vi "Periodic Tasks.vi"(8 "error in":errorcluster) -> ()   [LabVIEW 2013]
doc: "This VI runs in parallel to other tasks. It can contain as many user-defined periodic loops as you need. These can carry out PID or other sorts of timed response."
uses:
  <vilib>/Rock Robotics/SystemInterfaces/Utilities/FPGA_UtilitiesLED Source.ctl
  <vilib>/Rock Robotics/SystemInterfaces/Utilities/FPGA_UtilitiesLED State.ctl
  <vilib>/Rock Robotics/WPI/Solenoid/WPI_SolenoidValue.ctl
  Robot Global Data.vi
  <vilib>/Rock Robotics/WPI/Solenoid/WPI_SolenoidSetEnum.vi
  <vilib>/Rock Robotics/WPI/Compressor/WPI_CompressorGetSetRefNum.vi
  <vilib>/Rock Robotics/WPI/RobotDrive/WPI_RobotDriveGetSetRefNum.vi
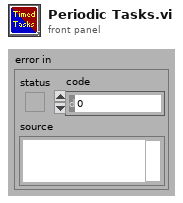
[diagram p1: front panel]
types:
  T1 = typedef "FPGA_UtilitiesLED State.ctl" = enum16{"Off", "On", "Toggle"}
  T2 = typedef "FPGA_UtilitiesLED Source.ctl" = enum16{"User LED", "FPGA LED"}
  T3 = typedef "WPI_CompressorDevRef.ctl" = cluster{"DevStatus":errorcluster, "DigitalInputDevRef":T4, "RelayDevRef":T7}
  T4 = typedef "WPI_DigitalInputDevRef.ctl" = cluster{"DevStatus":errorcluster, "DIO Channel":T5, "Digital Module":T6}
  T5 = typedef "FPGA_DIOChannel.ctl" = enum8{"DIO 1", "DIO 2", "DIO 3", "DIO 4", "DIO 5", "DIO 6", "DIO 7", "DIO 8", "DIO 9", "DIO 10", "DIO 11", "DIO 12", "DIO 13", "DIO 14", "Invalid"}
  T6 = typedef "FPGA_TypedefDigitalModule.ctl" = enum16{"Digital Module 1", "Digital Module 2"}
  T7 = typedef "WPI_RelayDevRef.ctl" = cluster{"DevStatus":errorcluster, "Relay Channel":T8, "Digital Module":T6, "Relay Direction":T9}
  T8 = typedef "FPGA_DIORelayChannel.ctl" = enum8{"Relay 1", "Relay 2", "Relay 3", "Relay 4", "Relay 5", "Relay 6", "Relay 7", "Relay 8", "Invalid"}
  T9 = typedef "WPI_RelayDirection.ctl" = enum16{"Both directions", "Forward only", "Reverse only"}
  T10 = typedef "WPI_RobotDriveDevRef.ctl" = cluster{"DevStatus":errorcluster, "Motors[]":T11[], "Square Inputs":bool, "Max Output":dbl, "Isochronous":bool}
  T11 = typedef "WPI_MotorControlDeviceRef.ctl" = cluster{"DeviceStatus":errorcluster, "Type":enum16{"PWM", "CAN"}, "PWM":cluster{"Digital Module":T6, "PWM Channel":T12, "DeadBand":T13}, "CAN":cluster{"Device Number":u8, "Control Mode":T14, "Semaphore":T15, "Max Vout":dbl}, "Invert":bool, "TransformRef":T16, "InvTransformRef":T16}
  T12 = typedef "FPGA_DIOPWMChannel.ctl" = enum8{"PWM 1", "PWM 2", "PWM 3", "PWM 4", "PWM 5", "PWM 6", "PWM 7", "PWM 8", "PWM 9", "PWM 10", "Invalid"}
  T13 = typedef "WPI_PWMDeadband.ctl" = cluster{"Name":string, "maxPositivePwm":i32, "minPositivePwm":i32, "centerPwm":i32, "maxNegativePwm":i32, "minNegativePwm":i32, "angularRange":u16}
  T14 = typedef "WPI_CANJaguar_ControlMode.ctl" = enum8{"Percent VBus", "Current", "Speed", "Position", "Voltage"}
  T15 = typedef "Semaphore RefNum" = refnum<k1>
  T16 = typedef "WPI_PWMTransform_ConPane.ctl" = refnum<vi>
  T17 = typedef "WPI_SolenoidDevRef.ctl" = cluster{"DevStatus":errorcluster, "Solenoid Module":T18, "Forward Solenoid Channel":T19, "Reverse Solenoid Channel":T19}
  T18 = typedef "FPGA_TypedefSolenoidModule.ctl" = enum16{"Solenoid Module 1", "Solenoid Module 2"}
  T19 = typedef "WPI_SolenoidChannel.ctl" = enum8{"Solenoid 1", "Solenoid 2", "Solenoid 3", "Solenoid 4", "Solenoid 5", "Solenoid 6", "Solenoid 7", "Solenoid 8", "Invalid"}
  T20 = cluster{"X-Axis":dbl, "Y-Axis":dbl, "Bottom Lever":dbl, "Trigger":bool, "Button 2":bool, "Button 3":bool, "Button 4":bool, "Button 5":bool, "Button 6":bool, "Button 7":bool, "Button 8":bool, "Button 9":bool, "Button 10":bool, "Button 11":bool}
  T21 = typedef "WPI_SolenoidValue.ctl" = enum16{"Off", "On", "Forward", "Reverse"}
  T22 = typedef "WPI_EncoderDevRef.ctl" = cluster{"DevStatus":errorcluster, "EncoderIndex":T23, "CounterIndex":T24, "DistancePerCount":dbl, "Decoding Type":T25}
  T23 = typedef "FPGA_EncoderIdx.ctl" = enum8{"Enc 0", "Enc 1", "Enc 2", "Enc 3", "Invalid"}
  T24 = typedef "FPGA_CounterCtrSystemIndex.ctl" = enum8{"Ctr 0", "Ctr 1", "Ctr 2", "Ctr 3", "Ctr 4", "Ctr 5", "Ctr 6", "Ctr 7", "Invalid"}
  T25 = typedef "WPI_EncoderType.ctl" = enum16{"1x", "2x", "4x"}
  T26 = typedef "WPI_DriverStationRobotMode2.ctl" = enum16{"Autonomous Disabled", "Autonomous Enabled", "Teleop Disabled", "Teleop Enabled", "Timeout", "Finish", "Test Disabled", "Test Enabled"}
  T27 = cluster{"Turret Angle":dbl, "Distance":dbl, "Crankback Auto?":bool, "Value":bool}
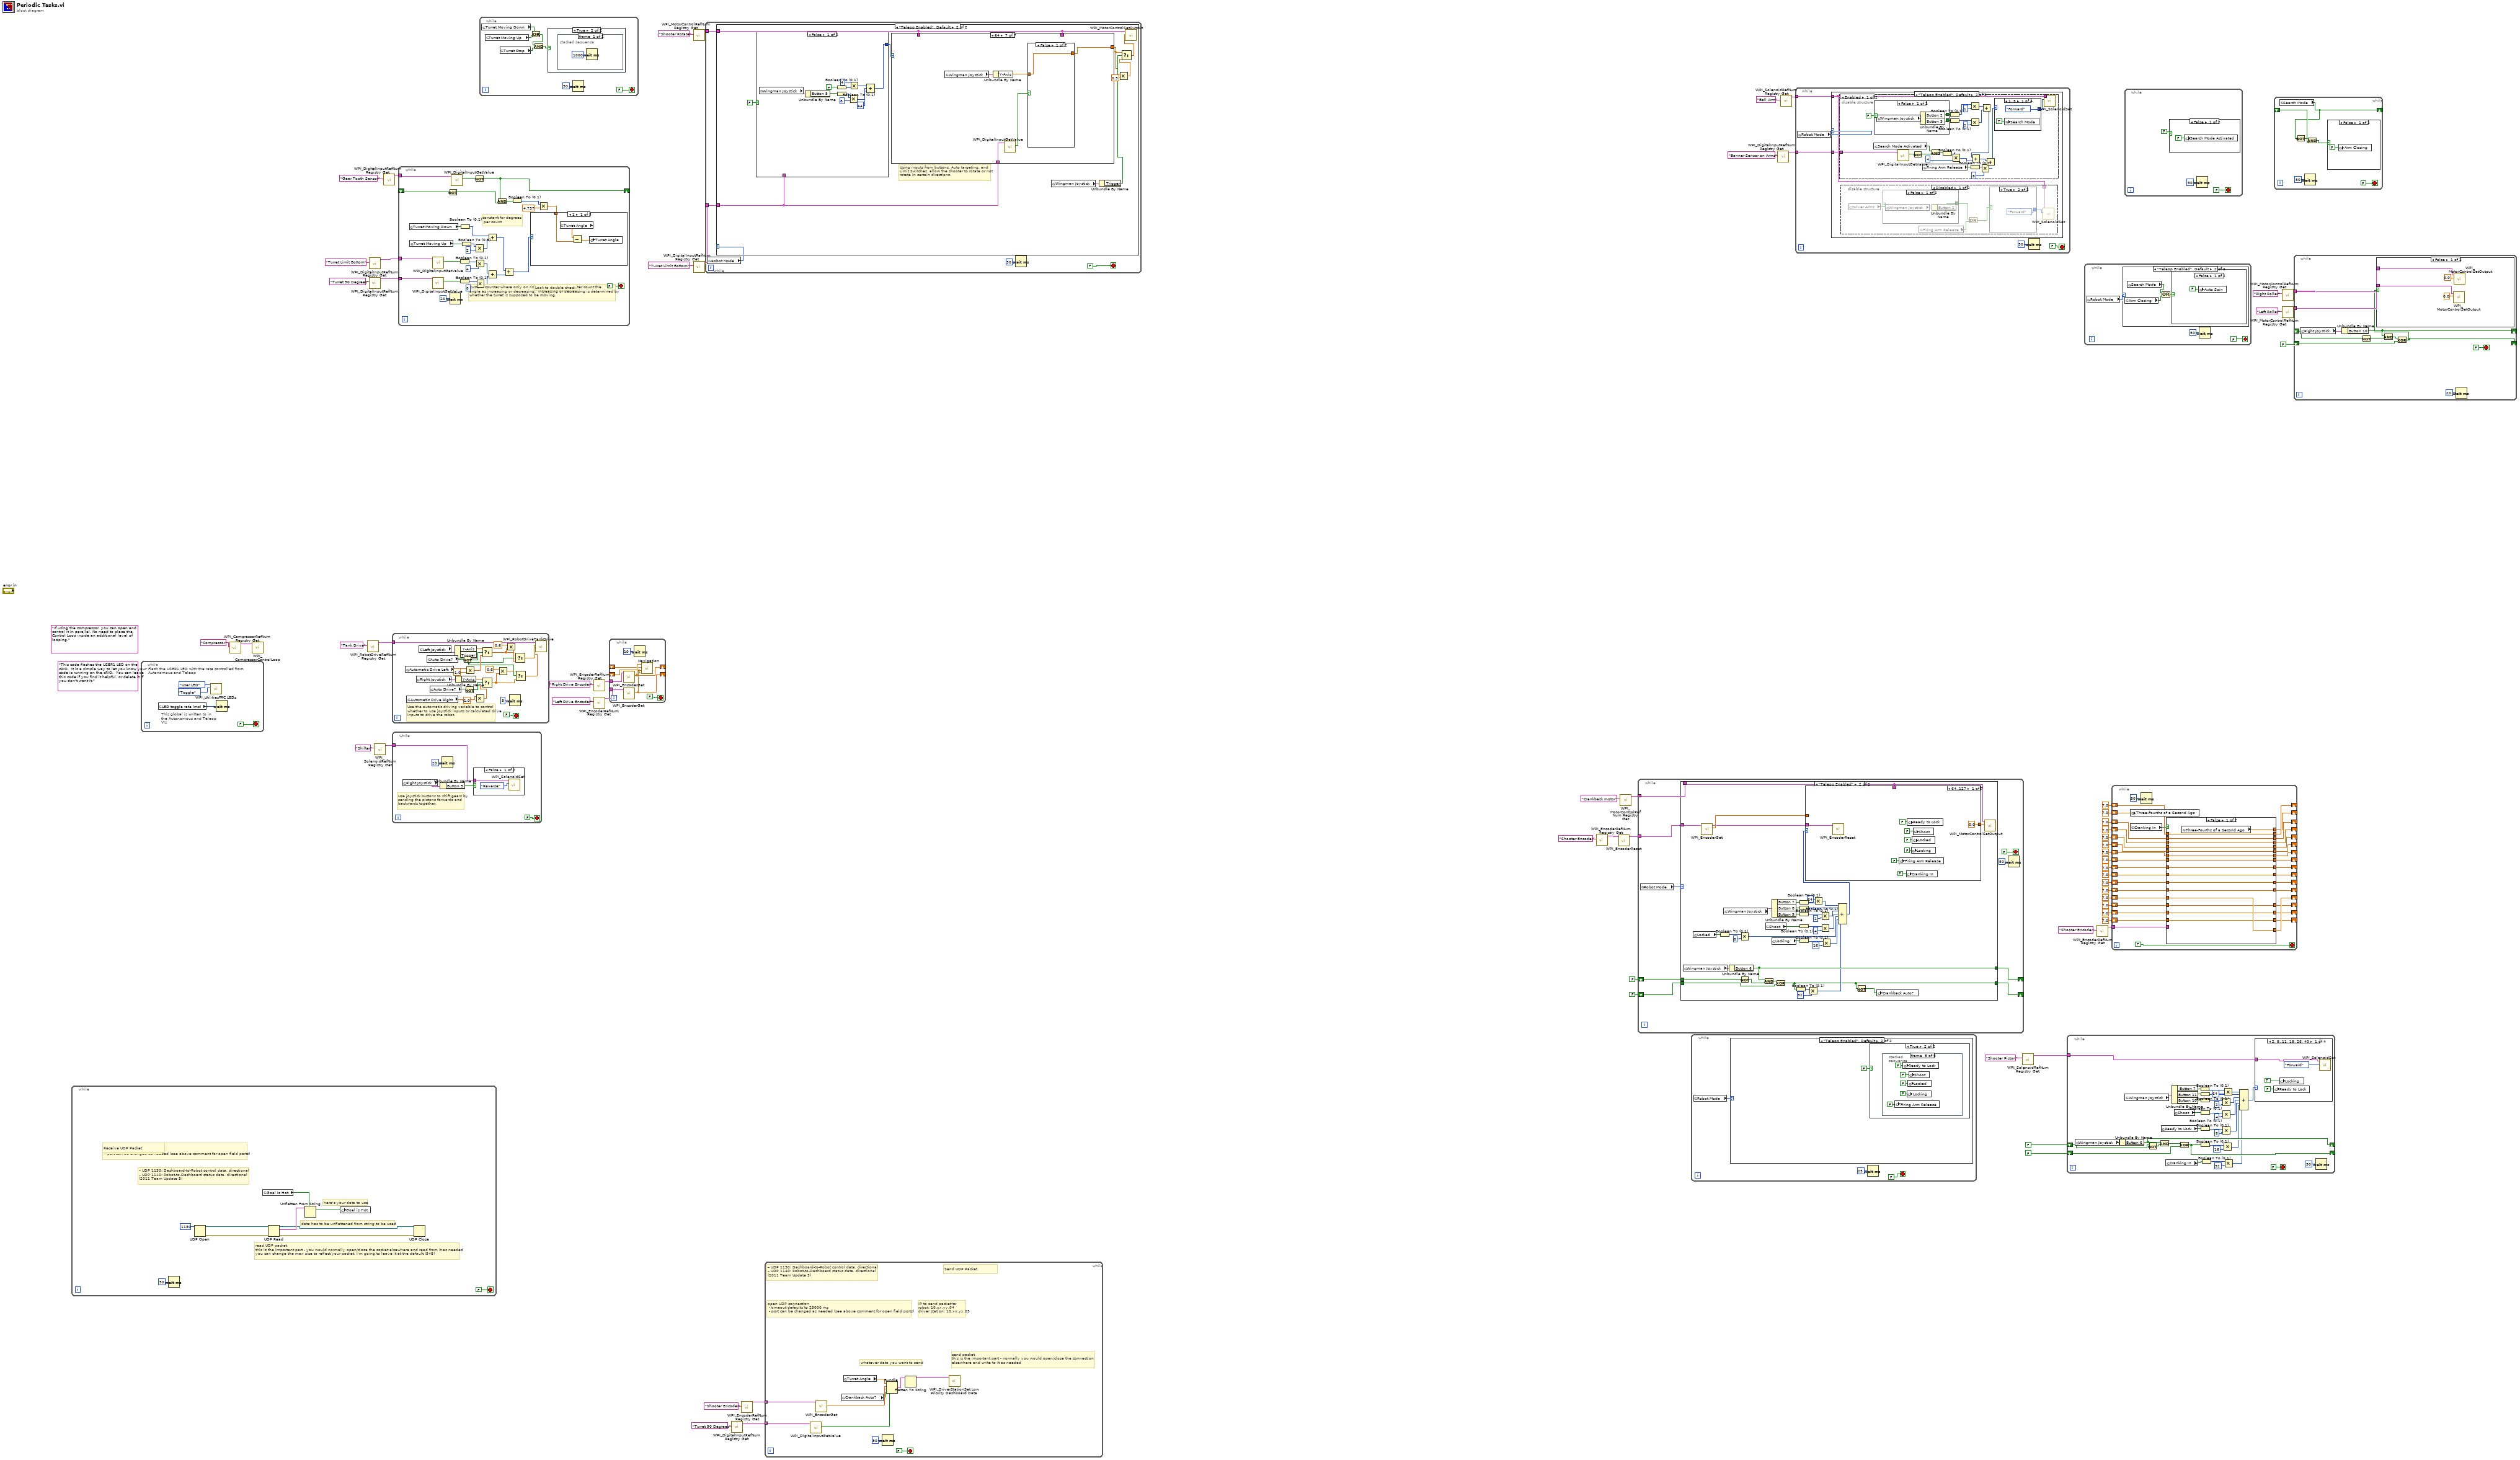
[diagram p0: block diagram]
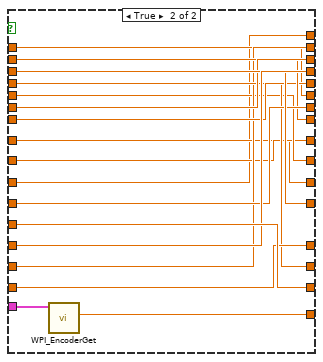
[diagram p2: hidden frame]
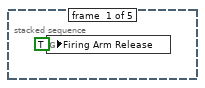
[diagram p5: hidden frame]
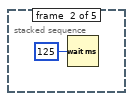
[diagram p6: hidden frame]
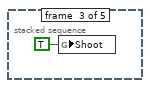
[diagram p7: hidden frame]
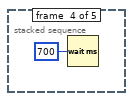
[diagram p8: hidden frame]
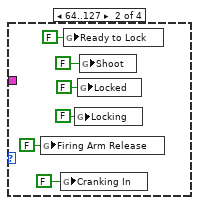
[diagram p9: hidden frame]
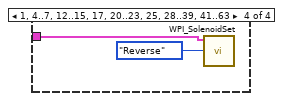
[diagram p11: hidden frame]
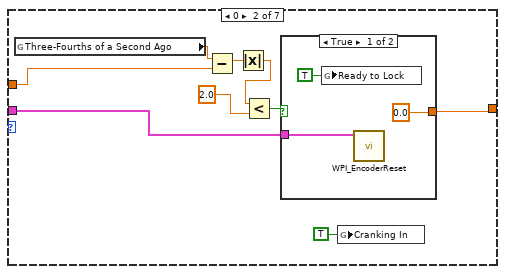
[diagram p13: hidden frame]
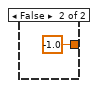
[diagram p14: hidden frame]
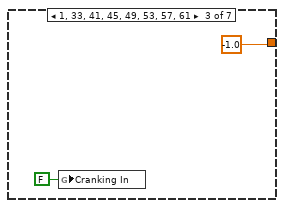
[diagram p15: hidden frame]
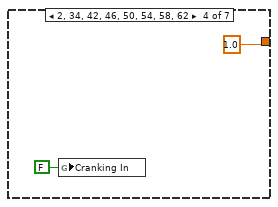
[diagram p16: hidden frame]
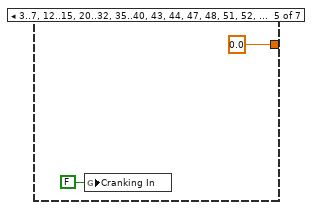
[diagram p17: hidden frame]
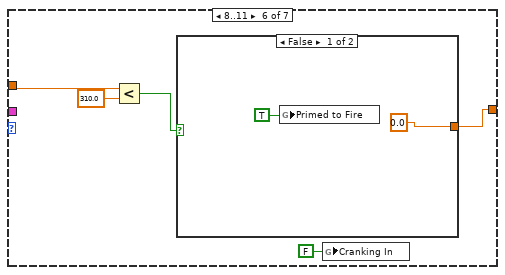
[diagram p18: hidden frame]
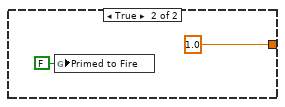
[diagram p19: hidden frame]
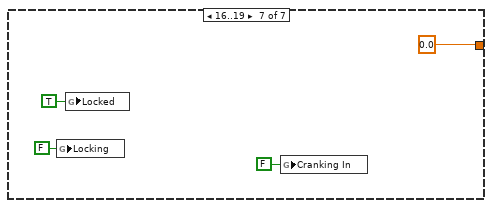
[diagram p20: hidden frame]
diagram:
  (unwired) "If using the compressor, you can open and control it in parallel. No need to place the Control Loop inside an additional level of looping."
  (unwired) "This code flashes the USER1 LED on the cRIO.  It is a simple way to let you know your code is running on the cRIO.  You can leave this code if you find it helpful, or delete it if you don't want it."
  n1 = while {
    stop <- FALSE stop-if-true
    # "here's your data to use"
    # "make sure that\nv  is the same as what you sent"
    # "data has to be unflattened from string to be used"
    # "read UDP packet\nthis is the important part - you would normally open/close the socket elsewhere and read from it as needed\nyou can change the max size to reflect your packet, I'm going to leave it at the default (548)"
    # "open UDP connection\n - timeout defaults to 25000 ms\n - port can be changed as needed (see above comment for open field ports)"
    # "– UDP 1130: Dashboard-to-Robot control data, directional\n– UDP 1140: Robot-to-Dashboard status data, directional\n(2011 Team Update 5)"
    # "Receive UDP Packet"
    n2 = Wait (ms)(milliseconds to wait=u32 50) -> ()  [unwired: 1 out]
    n3 = UDP Open(11:u16 1130 ("port")) -> (port=w69:refnum<k16>, 0:w68:errorcluster)  [unwired: 1 in, 4 out]
    n4 = global read "Robot Global Data.vi" "Goal is Hot"() -> (w64:bool)
    n5 = UDP Read(connection ID=w69, 8:w68) -> (data out=w67:string, error out=w65:errorcluster, 3:w66:refnum<k16>)  [unwired: 4 out]
    n6 = Unflatten From String(type=w64, binary string=w67) -> (value=w63:bool)  [unwired: 1 in, 4 out]
    n7 = global write "Robot Global Data.vi" "Goal is Hot"(w63) -> ()
    n8 = UDP Close(connection ID=w66, 8:w65) -> ()  [unwired: 2 out]
  }
  n9 = while {
    stop <- FALSE stop-if-true
    # "This global is written to in the Autonomous and Teleop VIs"
    # "Flash the USER1 LED with the rate controlled from Autonomous and Teleop"
    n10 = global read "Robot Global Data.vi" "LED toggle rate (ms)"() -> (w73:u32)
    n11 = call <vilib>:"WPI_UtilitiesFRC LEDs.vi"("State"=FPGA_UtilitiesLED_State."Toggle", "LED Type"=FPGA_UtilitiesLED_Source."User LED") -> ()  [unwired: 1 in, 9 out]
    n12 = Wait (ms)(milliseconds to wait=w73) -> ()  [unwired: 1 out]
  }
  n13 = call <vilib>:"WPI_CompressorRefNum Registry Get.vi"("refnum name"="Compressor") -> ("CompressorDevRef"=w58:T3)  [unwired: 9 in, 1 out]
  n14 = call <vilib>:"WPI_CompressorControlLoop.vi"("CompressorDevRef"=w58) -> ()  [unwired: 11 in]
  n15 = call <vilib>:"WPI_RobotDriveRefNum Registry Get.vi"("refnum name"="Tank Drive") -> ("RobotDriveDevRef"=w61:T10)  [unwired: 9 in, 1 out]
  n16 = call <vilib>:"WPI_DigitalInputRefNum Registry Get.vi"("refnum name"="Turret 90 Degrees") -> ("DigitalInputDevRef"=w35:T4)  [unwired: 9 in, 1 out]
  n17 = call <vilib>:"WPI_DigitalInputRefNum Registry Get.vi"("refnum name"="Turret Limit Bottom") -> ("DigitalInputDevRef"=w36:T4)  [unwired: 9 in, 1 out]
  n18 = call <vilib>:"WPI_SolenoidRefNum Registry Get.vi"("refnum name"="Shifter") -> ("SolenoidDevRef"=w60:T17)  [unwired: 9 in, 1 out]
  n19 = call <vilib>:"WPI_DigitalInputRefNum Registry Get.vi"("refnum name"="Gear Tooth Sensor") -> ("DigitalInputDevRef"=w39:T4)  [unwired: 9 in, 1 out]
  n20 = while {
    tunnel: w61 -> [w101]
    stop <- FALSE stop-if-true
    # "Use the automatic driving variable to control whether to use joystick inputs or calculated drive inputs to drive the robot."
    n21 = global read "Robot Global Data.vi" "Automatic Drive Left"() -> (w88:dbl)
    n22 = global read "Robot Global Data.vi" "Automatic Drive Right"() -> (w91:dbl)
    n23 = global read "Robot Global Data.vi" "Right Joystick"() -> (w97:T20)
    n24 = global read "Robot Global Data.vi" "Left Joystick"() -> (w99:T20)
    n25 = global read "Robot Global Data.vi" "Auto Drive?"() -> (w95:bool)
    n26 = global read "Robot Global Data.vi" "Auto Drive?"() -> (w93:bool)
    n27 = Unbundle By Name(w99) -> ("Y-Axis"=w98:dbl, "Trigger"=w81:bool)
    n28 = Unbundle By Name(w97) -> ("Y-Axis"=w96:dbl)
    n29 = Not(x=w95) -> (.not. x?=w94:bool)
    n30 = Not(x=w93) -> (.not. x?=w92:bool)
    n31 = Multiply(x=w88, y=-1.0) -> (x*y=w86:dbl)
    n32 = Multiply(x=w91, y=-1.0) -> (x*y=w89:dbl)
    n33 = Select(t=w98, s=w94, f=w86) -> (s? t:f=w84:dbl)
    n34 = Select(t=w96, s=w92, f=w89) -> (s? t:f=w79:dbl)
    n35 = Multiply(x=0.6, y=w79) -> (x*y=w80:dbl)
    n36 = Multiply(x=0.6, y=w84) -> (x*y=w83:dbl)
    n37 = Wait (ms)(milliseconds to wait=u32 5) -> ()  [unwired: 1 out]
    n38 = Select(t=w83, s=w81, f=w84) -> (s? t:f=w82:dbl)
    n39 = Select(t=w80, s=w81, f=w79) -> (s? t:f=w77:dbl)
    n40 = call <vilib>:"WPI_RobotDriveTankDrive.vi"("Right axis value"=w77, "Left axis value"=w82, "RobotDriveDevRef"=w101) -> ()  [unwired: 6 in, 3 out]
  }
  n41 = while {
    tunnel: w60 -> [w104]
    stop <- FALSE stop-if-true
    # "Use joystick buttons to shift gears by sending the pistons forwards and backwards together."
    n42 = global read "Robot Global Data.vi" "Right Joystick"() -> (w106:T20)
    n43 = Unbundle By Name(w106) -> ("Button 5"=w105:bool)
    n44 = Wait (ms)(milliseconds to wait=u32 20) -> ()  [unwired: 1 out]
    n45 = case shown="False" w105 {
      tunnel: w104 -> [w108 w111]
      frame False {
        n46 = call-poly <vilib>:"WPI_SolenoidSet.vi"("Value"=WPI_SolenoidValue."Reverse", "SolenoidDevRef"=w108) -> ()  [unwired: 8 in, 2 out]
      }
      frame True {
        n47 = call-poly <vilib>:"WPI_SolenoidSet.vi"("Value"=WPI_SolenoidValue."Forward", "SolenoidDevRef"=w111) -> ()  [unwired: 8 in, 2 out]
      }
    }
  }
  n48 = while {
    tunnel: w39 -> [w140]
    shift-right: [w127] -> _
    shift-left: _ -> [w138]
    tunnel: w36 -> [w125]
    tunnel: w35 -> [w124]
    stop <- FALSE stop-if-true
    # "Look to double check"
    # "Custom counter where only on rising edge will the counter count the\nangle as increasing or decreasing.  Increasing or decreasing is determined by \nwhether the turret is supposed to be moving."
    # "constant for degrees\n per count"
    n49 = global read "Robot Global Data.vi" "Turret Moving Down"() -> (w134:bool)
    n50 = global read "Robot Global Data.vi" "Turret Moving Up"() -> (w135:bool)
    n51 = call <vilib>:"WPI_DigitalInputGetValue.vi"("DigitalInputDevRef"=w124) -> ("Value"=w113:bool)  [unwired: 8 in, 2 out]
    n52 = call <vilib>:"WPI_DigitalInputGetValue.vi"("DigitalInputDevRef"=w125) -> ("Value"=w114:bool)  [unwired: 8 in, 2 out]
    n53 = Not(x=w138) -> (.not. x?=w137:bool)
    n54 = Wait (ms)(milliseconds to wait=u32 20) -> ()  [unwired: 1 out]
    n55 = call <vilib>:"WPI_DigitalInputGetValue.vi"("DigitalInputDevRef"=w140) -> ("Value"=w126:bool)  [unwired: 8 in, 2 out]
    n56 = Boolean To (0,1)(Boolean=w114) -> (0, 1=w123:i16)
    n57 = Boolean To (0,1)(Boolean=w113) -> (0, 1=w121:i16)
    n58 = Boolean To (0,1)(Boolean=w134) -> (0, 1=w131:i16)
    n59 = Boolean To (0,1)(Boolean=w135) -> (0, 1=w133:i16)
    n60 = Not(x=w126) -> (.not. x?=w127:bool)
    n61 = Multiply(x=w133, y=i16 2) -> (x*y=w130:i16)
    n62 = Multiply(x=w123, y=i16 4) -> (x*y=w118:i16)
    n63 = Multiply(x=w121, y=i16 8) -> (x*y=w119:i16)
    n64 = Add(x=w131, y=w130) -> (x+y=w116:i16)
    n65 = Add(x=w118, y=w119) -> (x+y=w117:i16)
    n66 = And(x=w127, y=w137) -> (x .and. y?=w136:bool)
    n67 = Add(x=w116, y=w117) -> (x+y=w115:i16)
    n68 = Boolean To (0,1)(Boolean=w136) -> (0, 1=w129:i16)
    n69 = Multiply(x=w129, y=4.737) -> (x*y=w128:dbl)
    n70 = case shown="1" w115 {
      tunnel: w128 -> [w142 w145 _ _ _]
      frame 1 {
        n71 = global read "Robot Global Data.vi" "Turret Angle"() -> (w143:dbl)
        n72 = Subtract(x=w143, y=w142) -> (x-y=w144:dbl)
        n73 = global write "Robot Global Data.vi" "Turret Angle"(w144) -> ()
      }
      frame 2 {
        n74 = global read "Robot Global Data.vi" "Turret Angle"() -> (w146:dbl)
        n75 = Add(x=w146, y=w145) -> (x+y=w147:dbl)
        n76 = global write "Robot Global Data.vi" "Turret Angle"(w147) -> ()
      }
      frame 4..7 {
        n77 = global write "Robot Global Data.vi" "Turret Angle"(0.0 ("Turret Angle")) -> ()
      }
      frame 8..11 {
        n78 = global write "Robot Global Data.vi" "Turret Angle"(90.0 ("Turret Angle")) -> ()
      }
      frame 0, 3, Default {
      }
    }
  }
  n79 = while {
    stop <- FALSE stop-if-true
    n80 = global read "Robot Global Data.vi" "Turret Moving Down"() -> (w153:bool)
    n81 = global read "Robot Global Data.vi" "Turret Moving Up"() -> (w154:bool)
    n82 = global read "Robot Global Data.vi" "Turret Stop"() -> (w150:bool)
    n83 = Or(x=w153, y=w154) -> (x .or. y?=w151:bool)
    n84 = And(x=w151, y=w150) -> (x .and. y?=w152:bool)
    n85 = case shown="True" w152 {
      frame False {
      }
      frame True {
        n86 = stacked-sequence {
          frame #0 {
            n87 = Wait (ms)(milliseconds to wait=u32 1000) -> ()  [unwired: 1 out]
          }
          frame #1 {
            n88 = global write "Robot Global Data.vi" "Turret Moving Down"(FALSE ("Turret Moving Down")) -> ()
            n89 = global write "Robot Global Data.vi" "Turret Moving Up"(FALSE ("Turret Moving Up")) -> ()
          }
        }
      }
    }
    n90 = Wait (ms)(milliseconds to wait=u32 50) -> ()  [unwired: 1 out]
  }
  n91 = call <vilib>:"WPI_EncoderRefNum Registry Get.vi"("refnum name"="Right Drive Encoder") -> ("EncoderDevRef"=w44:T22)  [unwired: 9 in, 1 out]
  n92 = call <vilib>:"WPI_EncoderRefNum Registry Get.vi"("refnum name"="Left Drive Encoder") -> ("EncoderDevRef"=w43:T22)  [unwired: 9 in, 1 out]
  n93 = while {
    tunnel: w44 -> [w167]
    tunnel: w43 -> [w166]
    shift-right: [w163] -> _
    shift-left: _ -> [w162]
    shift-right: [w161] -> _
    shift-left: _ -> [w160]
    stop <- FALSE stop-if-true
    n94 = call <vilib>:"WPI_EncoderGet.vi"("EncoderDevRef"=w167) -> ("Distance"=w163:dbl)  [unwired: 5 in, 5 out]
    n95 = call <vilib>:"WPI_EncoderGet.vi"("EncoderDevRef"=w166) -> ("Distance"=w161:dbl)  [unwired: 5 in, 5 out]
    n96 = Wait (ms)(milliseconds to wait=u32 10) -> ()  [unwired: 1 out]
    n97 = call "Navigation.vi"("Prev Left Encoder"=w160, "Left Encoder"=w161, "Prev Right Encoder"=w162, "Right Encoder"=w163) -> ()  [unwired: 8 in]
  }
  n98 = call <vilib>:"WPI_MotorControlRefNum Registry Get.vi"("refnum name"="Shooter Rotate") -> ("MotorControlDevRef"=w55:T11)  [unwired: 9 in, 1 out]
  n99 = call <vilib>:"WPI_DigitalInputRefNum Registry Get.vi"("refnum name"="Turret Limit Bottom") -> ("DigitalInputDevRef"=w53:T4)  [unwired: 9 in, 1 out]
  n100 = while {
    tunnel: w55 -> [w171]
    tunnel: w53 -> [w170]
    stop <- FALSE stop-if-true
    n101 = global read "Robot Global Data.vi" "Robot Mode"() -> (w168:T26)
    n102 = case shown="\"Teleop Enabled\", Default" w168 {
      tunnel: w171 -> [_ w180]
      tunnel: w170 -> [_ w181]
      frame "Autonomous Enabled" {
      }
      frame "Teleop Enabled", Default {
        # "Using inputs from buttons, Auto targeting, and Limit Switches, allow the shooter to rotate or not rotate in certain directions."
        n103 = case shown="False" FALSE {
          tunnel: w181 -> [_ w213]
          tunnel: [w185 w194] -> w182
          frame False {
            n104 = global read "Robot Global Data.vi" "Wingman Joystick"() -> (w193:T20)
            n105 = Unbundle By Name(w193) -> ("Button 5"=w184:bool)
            n106 = Boolean To (0,1)(Boolean=w184) -> (0, 1=w192:i16)
            n107 = Boolean To (0,1)(Boolean=FALSE) -> (0, 1=w190:i16)
            n108 = Multiply(x=w192, y=i16 8) -> (x*y=w187:i16)
            n109 = Multiply(x=i16 4, y=w190) -> (x*y=w188:i16)
            n110 = Compound Arithmetic op=ADD(w188, w187, i16 64 ("value")) -> (w185:i16)
          }
          frame True {
            n111 = global read "Robot Global Data.vi" "Left Joystick"() -> (w218:T20)
            n112 = Unbundle By Name(w218) -> ("Button 2"=w217:bool, "Button 3"=w216:bool, "Button 4"=w209:bool, "Button 5"=w208:bool, "Button 10"=w203:bool)
            n113 = call <vilib>:"WPI_DigitalInputGetValue.vi"("DigitalInputDevRef"=w213) -> ("Value"=w210:bool)  [unwired: 8 in, 2 out]
            n114 = Boolean To (0,1)(Boolean=w217) -> (0, 1=w200:i16)
            n115 = Boolean To (0,1)(Boolean=w216) -> (0, 1=w215:i16)
            n116 = Boolean To (0,1)(Boolean=w209) -> (0, 1=w204:i16)
            n117 = Boolean To (0,1)(Boolean=w208) -> (0, 1=w205:i16)
            n118 = Boolean To (0,1)(Boolean=w203) -> (0, 1=w202:i16)
            n119 = Boolean To (0,1)(Boolean=w210) -> (0, 1=w212:i16)
            n120 = Multiply(x=w215, y=i16 2) -> (x*y=w199:i16)
            n121 = Multiply(x=w204, y=i16 4) -> (x*y=w198:i16)
            n122 = Multiply(x=w205, y=i16 8) -> (x*y=w197:i16)
            n123 = Multiply(x=w202, y=i16 32) -> (x*y=w196:i16)
            n124 = Multiply(x=w212, y=i16 16) -> (x*y=w195:i16)
            n125 = Compound Arithmetic op=ADD(w200, w199, w198, w197, w196, w195) -> (w194:i16)
          }
        }
        n126 = case shown="64" w182 {
          tunnel: [0.0 -0.3 1.0 w227 w261 -1.0 w270] -> w174
          tunnel: w180 -> [_ _ _ w228 w262 _ _]
          tunnel: w181 -> [_ _ _ _ _ _ w271]
          tunnel: w180 -> [_ _ _ _ w260 _ _]
          frame 0, 3, 7, 11, 12, 15..17, 19, 21, 23, 25, 27..29, 31, Default {
            n127 = global write "Robot Global Data.vi" "Turret Stop"(TRUE ("Turret Moving Down")) -> ()
          }
          frame 1, 5, 9, 13 {
            n128 = global write "Robot Global Data.vi" "Turret Moving Down"(TRUE ("Turret Moving Down")) -> ()
            n129 = global write "Robot Global Data.vi" "Turret Moving Up"(FALSE ("Turret Moving Up")) -> ()
          }
          frame 2, 6, 10, 14, 18, 22, 26, 30 {
            n130 = global write "Robot Global Data.vi" "Turret Moving Down"(FALSE ("Turret Moving Down")) -> ()
            n131 = global write "Robot Global Data.vi" "Turret Moving Up"(TRUE ("Turret Moving Up")) -> ()
          }
          frame 4, 20, 68 {
            n132 = flat-sequence {
              tunnel: w228 -> [w229]
              tunnel: [0.0] -> w227
              frame #0 {
                n133 = while {
                  tunnel: w229 -> [w230]
                  stop <- w233 stop-if-true
                  n134 = global read "Robot Global Data.vi" "Turret Angle"() -> (w248:dbl)
                  n135 = global read "Robot Global Data.vi" "Turret Angle"() -> (w250:dbl)
                  n136 = global read "Robot Global Data.vi" "Left Joystick"() -> (w239:T20)
                  n137 = Less?(x=w250, y=90.0) -> (x < y?=w245:bool)
                  n138 = Greater?(x=w248, y=90.0) -> (0:w246:bool)
                  n139 = Wait (ms)(milliseconds to wait=u32 20) -> ()  [unwired: 1 out]
                  n140 = Unbundle By Name(w239) -> ("Button 2"=w238:bool, "Button 3"=w237:bool)
                  n141 = Boolean To (0,1)(Boolean=w246) -> (0, 1=w244:i16)
                  n142 = Boolean To (0,1)(Boolean=w245) -> (0, 1=w241:i16)
                  n143 = Multiply(x=w244, y=i16 2) -> (x*y=w242:i16)
                  n144 = Add(x=w241, y=w242) -> (x+y=w240:i16)
                  n145 = Or(x=w238, y=w237) -> (x .or. y?=w234:bool)
                  n146 = case shown="0, 3, Default" w240 {
                    tunnel: [0.0 1.0 -1.0] -> w231
                    frame 0, 3, Default {
                      n147 = global write "Robot Global Data.vi" "Turret Stop"(TRUE ("Turret Moving Down")) -> ()
                    }
                    frame 1 {
                      n148 = global write "Robot Global Data.vi" "Turret Moving Down"(FALSE ("Turret Moving Down")) -> ()
                      n149 = global write "Robot Global Data.vi" "Turret Moving Up"(TRUE ("Turret Moving Up")) -> ()
                    }
                    frame 2 {
                      n150 = global write "Robot Global Data.vi" "Turret Moving Down"(TRUE ("Turret Moving Down")) -> ()
                      n151 = global write "Robot Global Data.vi" "Turret Moving Up"(FALSE ("Turret Moving Up")) -> ()
                    }
                  }
                  n152 = Equal?(x=w231, y=0.0) -> (x = y?=w235:bool)
                  n153 = Or(x=w235, y=w234) -> (x .or. y?=w233:bool)
                  n154 = call <vilib>:"WPI_MotorControlSetOutput.vi"("Output"=w231, "MotorControlDevRef"=w230) -> ()  [unwired: 7 in, 3 out]
                }
              }
              frame #1 {
              }
            }
          }
          frame 8, 24, 72 {
            n155 = flat-sequence {
              tunnel: w262 -> [_]
              tunnel: w260 -> [w263]
              tunnel: [0.0] -> w261
              frame #0 {
                n156 = call <vilib>:"WPI_MotorControlSetOutput.vi"("Output"=-1.0, "MotorControlDevRef"=w263) -> ()  [unwired: 7 in, 3 out]
              }
              frame #1 {
                n157 = Wait (ms)(milliseconds to wait=u32 300) -> ()  [unwired: 1 out]
              }
              frame #2 {
              }
            }
          }
          frame 32..63 {
          }
          frame 64 {
            n158 = global read "Robot Global Data.vi" "Wingman Joystick"() -> (w272:T20)
            n159 = Unbundle By Name(w272) -> ("Y-Axis"=w269:dbl)
            n160 = call <vilib>:"WPI_DigitalInputGetValue.vi"("DigitalInputDevRef"=w271) -> ("Value"=w268:bool)  [unwired: 8 in, 2 out]
            n161 = case shown="False" w268 {
              tunnel: w269 -> [w273 w277]
              tunnel: [w273 w274] -> w270
              frame False {
              }
              frame True {
                n162 = In Range and Coerce(upper limit=0.0, x=w277, lower limit=1.0) -> (coerced(x)=w274:dbl)  [unwired: 1 out]
              }
            }
          }
        }
        n163 = global read "Robot Global Data.vi" "Wingman Joystick"() -> (w178:T20)
        n164 = Unbundle By Name(w178) -> ("Trigger"=w177:bool)
        n165 = Multiply(x=w174, y=0.5) -> (x*y=w176:dbl)
        n166 = Select(t=w174, s=w177, f=w176) -> (s? t:f=w173:dbl)
        n167 = call <vilib>:"WPI_MotorControlSetOutput.vi"("Output"=w173, "MotorControlDevRef"=w180) -> ()  [unwired: 7 in, 3 out]
      }
    }
    n168 = Wait (ms)(milliseconds to wait=u32 50) -> ()  [unwired: 1 out]
  }
  n169 = call <vilib>:"WPI_DigitalInputRefNum Registry Get.vi"("refnum name"="Turret 90 Degrees") -> ("DigitalInputDevRef"=w2:T4)  [unwired: 9 in, 1 out]
  n170 = call <vilib>:"WPI_EncoderRefNum Registry Get.vi"("refnum name"="Shooter Encoder") -> ("EncoderDevRef"=w22:T22)  [unwired: 9 in, 1 out]
  n171 = while {
    tunnel: w22 -> [w284]
    tunnel: w2 -> [w279]
    stop <- FALSE stop-if-true
    # "send packet\nthis is the important part - normally you would open/close the connection \nelsewhere and write to it as needed"
    # "whatever data you want to send"
    # "IP to send packet to \nrobot: 10.xx.yy.04\ndriver station: 10.xx.yy.05"
    # "open UDP connection\n - timeout defaults to 25000 ms\n - port can be changed as needed (see above comment for open field ports)"
    # "Send UDP Packet"
    # "– UDP 1130: Dashboard-to-Robot control data, directional\n– UDP 1140: Robot-to-Dashboard status data, directional\n(2011 Team Update 5)"
    n172 = call <vilib>:"WPI_DigitalInputGetValue.vi"("DigitalInputDevRef"=w279) -> ("Value"=w278:bool)  [unwired: 8 in, 2 out]
    n173 = call <vilib>:"WPI_EncoderGet.vi"("EncoderDevRef"=w284) -> ("Distance"=w282:dbl)  [unwired: 5 in, 5 out]
    n174 = global read "Robot Global Data.vi" "Crankback Auto?"() -> (w280:bool)
    n175 = global read "Robot Global Data.vi" "Turret Angle"() -> (w283:dbl)
    n176 = Wait (ms)(milliseconds to wait=u32 50) -> ()  [unwired: 1 out]
    n177 = Bundle("Turret Angle"=w283, "Distance"=w282, "Crankback Auto?"=w280, "Value"=w278) -> (w281:T27)  [unwired: 1 in]
    n178 = Flatten To String(anything=w281) -> (data string=w285:string)  [unwired: 1 in, 4 out]
    n179 = call <vilib>:"WPI_DriverStationSet Low Priority Dashboard Data.vi"("User Data"=w285) -> ()  [unwired: 10 in, 1 out]
  }
  n180 = call <vilib>:"WPI_EncoderRefNum Registry Get.vi"("refnum name"="Shooter Encoder") -> ("EncoderDevRef"=w26:T22)  [unwired: 9 in, 1 out]
  n181 = call <vilib>:"WPI_EncoderReset.vi"("EncoderDevRef"=w26) -> ("EncoderDevRef"=w25:T22)  [unwired: 9 in, 1 out]
  n182 = call <vilib>:"WPI_MotorControlRefNum Registry Get.vi"("refnum name"="Crankback motor") -> ("MotorControlDevRef"=w33:T11)  [unwired: 9 in, 1 out]
  n183 = while {
    tunnel: w33 -> [w292]
    tunnel: w25 -> [w296]
    shift-right: [w295] -> _
    shift-left: FALSE ("Button 11") -> [w294]
    shift-right: [w291] -> _
    shift-left: FALSE -> [w293]
    stop <- FALSE stop-if-true
    n184 = global read "Robot Global Data.vi" "Robot Mode"() -> (w290:T26)
    n185 = case shown="\"Teleop Enabled\"" w290 {
      tunnel: w296 -> [_ w332]
      tunnel: [w298 w324] -> w295
      tunnel: w294 -> [w298 w323]
      tunnel: w293 -> [w297 w320]
      tunnel: w292 -> [_ w306]
      tunnel: [w297 w300] -> w291
      frame "Autonomous Enabled", Default {
      }
      frame "Teleop Enabled" {
        n186 = global read "Robot Global Data.vi" "Wingman Joystick"() -> (w325:T20)
        n187 = global read "Robot Global Data.vi" "Locked"() -> (w328:bool)
        n188 = call <vilib>:"WPI_EncoderGet.vi"("EncoderDevRef"=w332) -> ("Distance"=w317:dbl, "EncoderDevRef"=w305:T22)  [unwired: 5 in, 4 out]
        n189 = Boolean To (0,1)(Boolean=w328) -> (0, 1=w327:i16)
        n190 = global read "Robot Global Data.vi" "Wingman Joystick"() -> (w338:T20)
        n191 = Unbundle By Name(w325) -> ("Button 6"=w324:bool)
        n192 = Multiply(x=w327, y=i16 8) -> (x*y=w310:i16)
        n193 = Not(x=w323) -> (.not. x?=w322:bool)
        n194 = And(x=w324, y=w322) -> (x .and. y?=w321:bool)
        n195 = global read "Robot Global Data.vi" "Shoot"() -> (w330:bool)
        n196 = Unbundle By Name(w338) -> ("Button 7"=w304:bool, "Button 8"=w337:bool, "Button 9"=w336:bool)
        n197 = global read "Robot Global Data.vi" "Locking"() -> (w316:bool)
        n198 = Exclusive Or(1:w320, 2:w321) -> (0:w300:bool)
        n199 = Boolean To (0,1)(Boolean=w300) -> (0, 1=w319:i16)
        n200 = Boolean To (0,1)(Boolean=w304) -> (0, 1=w303:i16)
        n201 = Boolean To (0,1)(Boolean=w337) -> (0, 1=w313:i16)
        n202 = Boolean To (0,1)(Boolean=w336) -> (0, 1=w335:i16)
        n203 = Boolean To (0,1)(Boolean=w330) -> (0, 1=w331:i16)
        n204 = Boolean To (0,1)(Boolean=w316) -> (0, 1=w315:i16)
        n205 = Multiply(x=w319, y=i16 32) -> (x*y=w308:i16)
        n206 = Multiply(x=i16 64, y=w303) -> (x*y=w301:i16)
        n207 = Multiply(x=w335, y=i16 2) -> (x*y=w312:i16)
        n208 = Multiply(x=w331, y=i16 4) -> (x*y=w311:i16)
        n209 = Multiply(x=w315, y=i16 16) -> (x*y=w309:i16)
        n210 = Compound Arithmetic op=ADD(w301, w313, w312, w311, w310, w309, w308) -> (w307:i16)
        n211 = case shown="64..127" w307 {
          tunnel: [0.0 w355 -1.0 1.0 0.0 w367 0.0] -> w333
          tunnel: w317 -> [_ w352 _ _ _ w370 _]
          tunnel: w306 -> [_ _ _ _ _ _ _]
          tunnel: w305 -> [w346 w353 _ _ _ _ _]
          frame 64..127 {
            n212 = call <vilib>:"WPI_EncoderReset.vi"("EncoderDevRef"=w346) -> ()  [unwired: 9 in, 2 out]
            n213 = global write "Robot Global Data.vi" "Firing Arm Release"(FALSE ("Primed to Fire")) -> ()
            n214 = global write "Robot Global Data.vi" "Cranking In"(FALSE ("Cranking In")) -> ()
            n215 = global write "Robot Global Data.vi" "Ready to Lock"(FALSE ("Shoot")) -> ()
            n216 = global write "Robot Global Data.vi" "Locking"(FALSE ("Shoot")) -> ()
            n217 = global write "Robot Global Data.vi" "Locked"(FALSE ("Shoot")) -> ()
            n218 = global write "Robot Global Data.vi" "Shoot"(FALSE ("Shoot")) -> ()
          }
          frame 0 {
            n219 = global read "Robot Global Data.vi" "Three-Fourths of a Second Ago"() -> (w354:dbl)
            n220 = Subtract(x=w354, y=w352) -> (x-y=w350:dbl)
            n221 = Absolute Value(x=w350) -> (abs(x)=w348:dbl)
            n222 = Less?(x=w348, y=2.0) -> (x < y?=w349:bool)
            n223 = case shown="True" w349 {
              tunnel: [0.0 -1.0] -> w355
              tunnel: w353 -> [w356 _]
              frame True {
                n224 = global write "Robot Global Data.vi" "Ready to Lock"(TRUE ("Ready to Lock")) -> ()
                n225 = call <vilib>:"WPI_EncoderReset.vi"("EncoderDevRef"=w356) -> ()  [unwired: 9 in, 2 out]
              }
              frame False {
              }
            }
            n226 = global write "Robot Global Data.vi" "Cranking In"(TRUE ("Cranking In")) -> ()
          }
          frame 1, 33, 41, 45, 49, 53, 57, 61 {
            n227 = global write "Robot Global Data.vi" "Cranking In"(FALSE ("Cranking In")) -> ()
          }
          frame 2, 34, 42, 46, 50, 54, 58, 62 {
            n228 = global write "Robot Global Data.vi" "Cranking In"(FALSE ("Cranking In")) -> ()
          }
          frame 3..7, 12..15, 20..32, 35..40, 43, 44, 47, 48, 51, 52, 55, 56, 59, 60, 63, Default {
            n229 = global write "Robot Global Data.vi" "Cranking In"(FALSE ("Cranking In")) -> ()
          }
          frame 8..11 {
            n230 = Less?(x=w370, y=310.0) -> (x < y?=w368:bool)
            n231 = case shown="False" w368 {
              tunnel: [0.0 1.0] -> w367
              frame False {
                n232 = global write "Robot Global Data.vi" "Primed to Fire"(TRUE ("Locked")) -> ()
              }
              frame True {
                n233 = global write "Robot Global Data.vi" "Primed to Fire"(FALSE ("Locked")) -> ()
              }
            }
            n234 = global write "Robot Global Data.vi" "Cranking In"(FALSE ("Cranking In")) -> ()
          }
          frame 16..19 {
            n235 = global write "Robot Global Data.vi" "Locking"(FALSE ("Locked")) -> ()
            n236 = global write "Robot Global Data.vi" "Locked"(TRUE ("Locked")) -> ()
            n237 = global write "Robot Global Data.vi" "Cranking In"(FALSE ("Cranking In")) -> ()
          }
        }
        n238 = Not(x=w300) -> (.not. x?=w299:bool)
        n239 = global write "Robot Global Data.vi" "Crankback Auto?"(w299) -> ()
        n240 = call <vilib>:"WPI_MotorControlSetOutput.vi"("Output"=w333, "MotorControlDevRef"=w306) -> ()  [unwired: 7 in, 3 out]
      }
    }
    n241 = Wait (ms)(milliseconds to wait=u32 50) -> ()  [unwired: 1 out]
  }
  n242 = while {
    stop <- FALSE stop-if-true
    n243 = global read "Robot Global Data.vi" "Robot Mode"() -> (w379:T26)
    n244 = case shown="\"Teleop Enabled\", Default" w379 {
      frame "Autonomous Enabled" {
      }
      frame "Teleop Enabled", Default {
        n245 = case shown="True" FALSE {
          frame False {
          }
          frame True {
            n246 = stacked-sequence {
              frame #0 {
                n247 = global write "Robot Global Data.vi" "Firing Arm Release"(TRUE ("Primed to Fire")) -> ()
              }
              frame #1 {
                n248 = Wait (ms)(milliseconds to wait=u32 125) -> ()  [unwired: 1 out]
              }
              frame #2 {
                n249 = global write "Robot Global Data.vi" "Shoot"(TRUE ("Shoot")) -> ()
              }
              frame #3 {
                n250 = Wait (ms)(milliseconds to wait=u32 700) -> ()  [unwired: 1 out]
              }
              frame #4 {
                n251 = global write "Robot Global Data.vi" "Firing Arm Release"(FALSE ("Primed to Fire")) -> ()
                n252 = global write "Robot Global Data.vi" "Ready to Lock"(FALSE ("Shoot")) -> ()
                n253 = global write "Robot Global Data.vi" "Locking"(FALSE ("Shoot")) -> ()
                n254 = global write "Robot Global Data.vi" "Locked"(FALSE ("Shoot")) -> ()
                n255 = global write "Robot Global Data.vi" "Shoot"(FALSE ("Shoot")) -> ()
              }
            }
          }
        }
      }
    }
    n256 = Wait (ms)(milliseconds to wait=u32 25) -> ()  [unwired: 1 out]
  }
  n257 = call <vilib>:"WPI_DigitalInputRefNum Registry Get.vi"("refnum name"="Banner Sensor on Arms") -> ("DigitalInputDevRef"=w41:T4)  [unwired: 9 in, 1 out]
  n258 = call <vilib>:"WPI_SolenoidRefNum Registry Get.vi"("refnum name"="Ball Arm") -> ("SolenoidDevRef"=w51:T17)  [unwired: 9 in, 1 out]
  n259 = while {
    tunnel: w51 -> [w394]
    tunnel: w41 -> [w393]
    stop <- FALSE stop-if-true
    n260 = global read "Robot Global Data.vi" "Robot Mode"() -> (w392:T26)
    n261 = case shown="\"Teleop Enabled\", Default" w392 {
      tunnel: w394 -> [w397 w413]
      tunnel: w393 -> [_ w414]
      frame "Autonomous Enabled" {
        n262 = global read "Robot Global Data.vi" "Auto Arms Close"() -> (w406:bool)
        n263 = global read "Robot Global Data.vi" "Auto Arms Open"() -> (w407:bool)
        n264 = global read "Robot Global Data.vi" "Firing Arm Release"() -> (w408:bool)
        n265 = Boolean To (0,1)(Boolean=w406) -> (0, 1=w404:i16)
        n266 = Boolean To (0,1)(Boolean=w407) -> (0, 1=w405:i16)
        n267 = Boolean To (0,1)(Boolean=w408) -> (0, 1=w401:i16)
        n268 = Multiply(x=w405, y=i16 2) -> (x*y=w400:i16)
        n269 = Multiply(x=w404, y=i16 4) -> (x*y=w399:i16)
        n270 = Compound Arithmetic op=ADD(w401, w400, w399) -> (w398:i16)
        n271 = case shown="4" w398 {
          tunnel: w397 -> [w409 _ w411]
          frame 4 {
            n272 = call-poly <vilib>:"WPI_SolenoidSet.vi"("Value"=WPI_SolenoidValue."Reverse", "SolenoidDevRef"=w409) -> ()  [unwired: 8 in, 2 out]
          }
          frame 0, Default {
          }
          frame 1..3 {
            n273 = call-poly <vilib>:"WPI_SolenoidSet.vi"("Value"=WPI_SolenoidValue."Forward", "SolenoidDevRef"=w411) -> ()  [unwired: 8 in, 2 out]
          }
        }
      }
      frame "Teleop Enabled", Default {
        n274 = disable-structure shown="Enabled" {
          disable-tunnel: w413 -> [w452 _]
          disable-tunnel: w414 -> [w443 _]
          frame Enabled {
            n275 = global read "Robot Global Data.vi" "Search Mode Activated"() -> (w435:bool)
            n276 = case shown="False" FALSE {
              tunnel: [w453 w457] -> w445
              tunnel: [w454 w456] -> w444
              frame False {
                n277 = global read "Robot Global Data.vi" "Wingman Joystick"() -> (w455:T20)
                n278 = Unbundle By Name(w455) -> ("Button 2"=w454:bool, "Button 3"=w453:bool)
              }
              frame True {
                n279 = global read "Robot Global Data.vi" "Right Joystick"() -> (w458:T20)
                n280 = Unbundle By Name(w458) -> ("Button 2"=w456:bool, "Button 3"=w457:bool)
              }
            }
            n281 = call <vilib>:"WPI_DigitalInputGetValue.vi"("DigitalInputDevRef"=w443) -> ("Value"=w441:bool)  [unwired: 8 in, 2 out]
            n282 = Not(x=w441) -> (.not. x?=w434:bool)
            n283 = global read "Robot Global Data.vi" "Firing Arm Release"() -> (w440:bool)
            n284 = And(x=w435, y=w434) -> (x .and. y?=w433:bool)
            n285 = Boolean To (0,1)(Boolean=w433) -> (0, 1=w432:i16)
            n286 = Boolean To (0,1)(Boolean=w444) -> (0, 1=w451:i16)
            n287 = Boolean To (0,1)(Boolean=w445) -> (0, 1=w450:i16)
            n288 = Multiply(x=w432, y=i16 4) -> (x*y=w428:i16)
            n289 = Multiply(x=w451, y=i16 1) -> (x*y=w449:i16)
            n290 = Multiply(x=w450, y=i16 2) -> (x*y=w448:i16)
            n291 = Boolean To (0,1)(Boolean=w440) -> (0, 1=w438:i16)
            n292 = Multiply(x=w438, y=i16 8) -> (x*y=w437:i16)
            n293 = Add(x=w449, y=w448) -> (x+y=w429:i16)
            n294 = Add(x=w429, y=w428) -> (x+y=w430:i16)
            n295 = Add(x=w430, y=w437) -> (x+y=w439:i16)
            n296 = case shown="1, 5" w439 {
              tunnel: [WPI_SolenoidValue."Forward" ("Value") WPI_SolenoidValue."Reverse" ("Value") WPI_SolenoidValue."Forward" ("Value") WPI_SolenoidValue."Off" ("Value")] -> w442
              frame 1, 5 {
                n297 = global write "Robot Global Data.vi" "Search Mode"(TRUE ("Search Mode")) -> ()
              }
              frame 2, 4, 6 {
                n298 = global write "Robot Global Data.vi" "Search Mode"(FALSE ("Search Mode")) -> ()
              }
              frame 8..15 {
              }
              frame 0, 3, 7, Default {
              }
            }
            n299 = call-poly <vilib>:"WPI_SolenoidSet.vi"("Value"=w442, "SolenoidDevRef"=w452) -> ()  [unwired: 8 in, 2 out]
          }
          frame Disabled {
          }
        }
        n300 = disable-structure shown="Disabled" {
          disable-tunnel: w413 -> [w415 _]
          frame Disabled {
            n301 = global read "Robot Global Data.vi" "Driver Arms"() -> (w420:bool)
            n302 = case shown="False" w420 {
              tunnel: [w423 w425] -> w418
              frame False {
                n303 = global read "Robot Global Data.vi" "Wingman Joystick"() -> (w424:T20)
                n304 = Unbundle By Name(w424) -> ("Button 2"=w423:bool)
              }
              frame True {
                n305 = global read "Robot Global Data.vi" "Right Joystick"() -> (w426:T20)
                n306 = Unbundle By Name(w426) -> ("Button 2"=w425:bool)
              }
            }
            n307 = global read "Robot Global Data.vi" "Firing Arm Release"() -> (w419:bool)
            n308 = Or(x=w418, y=w419) -> (x .or. y?=w417:bool)
            n309 = case shown="True" w417 {
              tunnel: [WPI_SolenoidValue."Reverse" ("Value") WPI_SolenoidValue."Forward" ("Value")] -> w416
              frame False {
              }
              frame True {
              }
            }
            n310 = call-poly <vilib>:"WPI_SolenoidSet.vi"("Value"=w416, "SolenoidDevRef"=w415) -> ()  [unwired: 8 in, 2 out]
          }
          frame Enabled {
          }
        }
      }
    }
    n311 = Wait (ms)(milliseconds to wait=u32 50) -> ()  [unwired: 1 out]
  }
  n312 = call <vilib>:"WPI_SolenoidRefNum Registry Get.vi"("refnum name"="Shooter Piston") -> ("SolenoidDevRef"=w30:T17)  [unwired: 9 in, 1 out]
  n313 = while {
    tunnel: w30 -> [w494]
    shift-right: [w480] -> _
    shift-left: FALSE ("Button 11") -> [w481]
    shift-right: [w476] -> _
    shift-left: FALSE -> [w477]
    stop <- FALSE stop-if-true
    n314 = global read "Robot Global Data.vi" "Wingman Joystick"() -> (w493:T20)
    n315 = Unbundle By Name(w493) -> ("Button 6"=w480:bool)
    n316 = global read "Robot Global Data.vi" "Wingman Joystick"() -> (w499:T20)
    n317 = Not(x=w481) -> (.not. x?=w479:bool)
    n318 = And(x=w480, y=w479) -> (x .and. y?=w478:bool)
    n319 = global read "Robot Global Data.vi" "Ready to Lock"() -> (w489:bool)
    n320 = global read "Robot Global Data.vi" "Cranking In"() -> (w470:bool)
    n321 = Unbundle By Name(w499) -> ("Button 7"=w468:bool, "Button 11"=w498:bool, "Button 10"=w497:bool)
    n322 = global read "Robot Global Data.vi" "Shoot"() -> (w485:bool)
    n323 = Exclusive Or(1:w477, 2:w478) -> (0:w476:bool)
    n324 = Boolean To (0,1)(Boolean=w468) -> (0, 1=w467:i16)
    n325 = Boolean To (0,1)(Boolean=w498) -> (0, 1=w491:i16)
    n326 = Boolean To (0,1)(Boolean=w497) -> (0, 1=w496:i16)
    n327 = Boolean To (0,1)(Boolean=w485) -> (0, 1=w486:i16)
    n328 = Boolean To (0,1)(Boolean=w489) -> (0, 1=w488:i16)
    n329 = Boolean To (0,1)(Boolean=w476) -> (0, 1=w475:i16)
    n330 = Boolean To (0,1)(Boolean=w470) -> (0, 1=w472:i16)
    n331 = Multiply(x=w496, y=i16 2) -> (x*y=w490:i16)
    n332 = Multiply(x=w486, y=i16 4) -> (x*y=w483:i16)
    n333 = Multiply(x=w488, y=i16 8) -> (x*y=w482:i16)
    n334 = Multiply(x=w475, y=i16 16) -> (x*y=w473:i16)
    n335 = Multiply(x=w467, y=i16 64) -> (x*y=w465:i16)
    n336 = Multiply(x=w472, y=i16 32) -> (x*y=w469:i16)
    n337 = Compound Arithmetic op=ADD(w465, w491, w490, w483, w482, w473, w469) -> (w492:i16)
    n338 = case shown="2, 8..11, 18, 26, 40" w492 {
      tunnel: w494 -> [w504 _ _ w512]
      frame 2, 8..11, 18, 26, 40 {
        n339 = global write "Robot Global Data.vi" "Ready to Lock"(FALSE ("Ready to Lock")) -> ()
        n340 = global write "Robot Global Data.vi" "Locking"(TRUE ("Ready to Lock")) -> ()
        n341 = call-poly <vilib>:"WPI_SolenoidSet.vi"("Value"=WPI_SolenoidValue."Forward", "SolenoidDevRef"=w504) -> ()  [unwired: 8 in, 2 out]
      }
      frame 64..127 {
        n342 = global write "Robot Global Data.vi" "Firing Arm Release"(FALSE ("Primed to Fire")) -> ()
        n343 = global write "Robot Global Data.vi" "Cranking In"(FALSE ("Cranking In")) -> ()
        n344 = global write "Robot Global Data.vi" "Ready to Lock"(FALSE ("Shoot")) -> ()
        n345 = global write "Robot Global Data.vi" "Locking"(FALSE ("Shoot")) -> ()
        n346 = global write "Robot Global Data.vi" "Locked"(FALSE ("Shoot")) -> ()
        n347 = global write "Robot Global Data.vi" "Shoot"(FALSE ("Shoot")) -> ()
      }
      frame 0, 3, 16, 19, 24, 27, Default {
      }
      frame 1, 4..7, 12..15, 17, 20..23, 25, 28..39, 41..63 {
        n348 = call-poly <vilib>:"WPI_SolenoidSet.vi"("Value"=WPI_SolenoidValue."Reverse", "SolenoidDevRef"=w512) -> ()  [unwired: 8 in, 2 out]
      }
    }
    n349 = Wait (ms)(milliseconds to wait=u32 50) -> ()  [unwired: 1 out]
  }
  n350 = while {
    stop <- FALSE stop-if-true
    n351 = global read "Robot Global Data.vi" "Robot Mode"() -> (w514:T26)
    n352 = case shown="\"Teleop Enabled\", Default" w514 {
      frame "Autonomous Enabled" {
      }
      frame "Teleop Enabled", Default {
        n353 = global read "Robot Global Data.vi" "Arm Closing"() -> (w517:bool)
        n354 = global read "Robot Global Data.vi" "Search Mode"() -> (w518:bool)
        n355 = Or(x=w518, y=w517) -> (x .or. y?=w519:bool)
        n356 = case shown="False" w519 {
          frame False {
            n357 = global write "Robot Global Data.vi" "Auto Spin"(FALSE ("Auto Spin")) -> ()
          }
          frame True {
            n358 = global write "Robot Global Data.vi" "Auto Spin"(TRUE ("Auto Spin")) -> ()
          }
        }
      }
    }
    n359 = Wait (ms)(milliseconds to wait=u32 50) -> ()  [unwired: 1 out]
  }
  n360 = call <vilib>:"WPI_EncoderRefNum Registry Get.vi"("refnum name"="Shooter Encoder") -> ("EncoderDevRef"=w20:T22)  [unwired: 9 in, 1 out]
  n361 = while {
    tunnel: w20 -> [w555]
    shift-right: [w553] -> _
    shift-left: 7.0 ("Distance") -> [w552]
    shift-right: [w551] -> _
    shift-left: 7.0 ("Distance") -> [w550]
    shift-right: [w549] -> _
    shift-left: 7.0 ("Distance") -> [w548]
    shift-right: [w547] -> _
    shift-left: 7.0 ("Distance") -> [w546]
    shift-right: [w545] -> _
    shift-left: 7.0 ("Distance") -> [w544]
    shift-right: [w543] -> _
    shift-left: 7.0 ("Distance") -> [w541]
    shift-right: [w542] -> _
    shift-left: 7.0 ("Distance") -> [w540]
    shift-right: [w539] -> _
    shift-left: 7.0 ("Distance") -> [w537]
    shift-right: [w538] -> _
    shift-left: 7.0 ("Distance") -> [w536]
    shift-right: [w535] -> _
    shift-left: 7.0 ("Distance") -> [w533]
    shift-right: [w534] -> _
    shift-left: 7.0 ("Distance") -> [w531]
    shift-right: [w532] -> _
    shift-left: 7.0 ("Distance") -> [w529]
    shift-right: [w530] -> _
    shift-left: 7.0 ("Distance") -> [w528]
    shift-right: [w527] -> _
    shift-left: 7.0 ("Distance") -> [w526]
    shift-right: [w525] -> _
    shift-left: 7.0 ("Distance") -> [w524]
    shift-right: [w523] -> _
    shift-left: 7.0 ("Distance") -> [w522]
    stop <- FALSE stop-if-true
    n362 = global write "Robot Global Data.vi" "Three-Fourths of a Second Ago"(w522) -> ()
    n363 = global read "Robot Global Data.vi" "Cranking In"() -> (w554:bool)
    n364 = Wait (ms)(milliseconds to wait=u32 50) -> ()  [unwired: 1 out]
    n365 = case shown="False" w554 {
      tunnel: w555 -> [_ w590]
      tunnel: [w573 w589] -> w553
      tunnel: w552 -> [w573 w588]
      tunnel: [w572 w588] -> w551
      tunnel: w550 -> [w572 w587]
      tunnel: [w571 w587] -> w549
      tunnel: w548 -> [w571 w586]
      tunnel: [w570 w586] -> w547
      tunnel: w546 -> [w570 w585]
      tunnel: [w569 w585] -> w545
      tunnel: w544 -> [w569 w584]
      tunnel: [w568 w584] -> w543
      tunnel: [w567 w583] -> w542
      tunnel: w541 -> [w568 w583]
      tunnel: w540 -> [w567 w582]
      tunnel: [w566 w582] -> w539
      tunnel: [w565 w581] -> w538
      tunnel: w537 -> [w566 w581]
      tunnel: w536 -> [w565 w580]
      tunnel: [w564 w580] -> w535
      tunnel: [w563 w579] -> w534
      tunnel: w533 -> [w564 w579]
      tunnel: [w562 w578] -> w532
      tunnel: w531 -> [w563 w578]
      tunnel: [w561 w577] -> w530
      tunnel: w529 -> [w562 w577]
      tunnel: w528 -> [w561 w576]
      tunnel: [w560 w576] -> w527
      tunnel: w526 -> [w560 w575]
      tunnel: [w559 w575] -> w525
      tunnel: w524 -> [w559 w574]
      tunnel: [w558 w574] -> w523
      frame False {
        n366 = global read "Robot Global Data.vi" "Three-Fourths of a Second Ago"() -> (w558:dbl)
      }
      frame True {
        n367 = call <vilib>:"WPI_EncoderGet.vi"("EncoderDevRef"=w590) -> ("Distance"=w589:dbl)  [unwired: 5 in, 5 out]
      }
    }
  }
  n368 = while {
    stop <- FALSE stop-if-true
    n369 = case shown="False" FALSE {
      frame False {
        n370 = global write "Robot Global Data.vi" "Search Mode Activated"(FALSE ("Search Mode Activated")) -> ()
      }
      frame True {
        n371 = stacked-sequence {
          frame #0 {
            n372 = Wait (ms)(milliseconds to wait=u32 1000) -> ()  [unwired: 1 out]
          }
          frame #1 {
            n373 = global write "Robot Global Data.vi" "Search Mode Activated"(TRUE ("Search Mode Activated")) -> ()
          }
        }
      }
    }
    n374 = Wait (ms)(milliseconds to wait=u32 50) -> ()  [unwired: 1 out]
  }
  n375 = while {
    shift-right: [w599] -> _
    shift-left: _ -> [w600]
    stop <- FALSE stop-if-true
    n376 = global read "Robot Global Data.vi" "Search Mode"() -> (w599:bool)
    n377 = Not(x=w599) -> (.not. x?=w602:bool)
    n378 = Wait (ms)(milliseconds to wait=u32 50) -> ()  [unwired: 1 out]
    n379 = And(x=w602, y=w600) -> (x .and. y?=w601:bool)
    n380 = case shown="False" w601 {
      frame False {
        n381 = global write "Robot Global Data.vi" "Arm Closing"(FALSE ("Arm Closing")) -> ()
      }
      frame True {
        n382 = stacked-sequence {
          frame #0 {
            n383 = global write "Robot Global Data.vi" "Arm Closing"(TRUE ("Arm Closing")) -> ()
          }
          frame #1 {
            n384 = Wait (ms)(milliseconds to wait=u32 1000) -> ()  [unwired: 1 out]
          }
          frame #2 {
            n385 = global write "Robot Global Data.vi" "Arm Closing"(FALSE ("Arm Closing")) -> ()
          }
        }
      }
    }
  }
  n386 = call <vilib>:"WPI_MotorControlRefNum Registry Get.vi"("refnum name"="Right Roller") -> ("MotorControlDevRef"=w47:T11)  [unwired: 9 in, 1 out]
  n387 = call <vilib>:"WPI_MotorControlRefNum Registry Get.vi"("refnum name"="Left Roller") -> ("MotorControlDevRef"=w48:T11)  [unwired: 9 in, 1 out]
  n388 = while {
    tunnel: w48 -> [w616]
    tunnel: w47 -> [w615]
    shift-right: [w612] -> _
    shift-left: _ -> [w610]
    shift-right: [w608] -> _
    shift-left: FALSE -> [w607]
    stop <- FALSE stop-if-true
    n389 = global read "Robot Global Data.vi" "Right Joystick"() -> (w613:T20)
    n390 = Unbundle By Name(w613) -> ("Button 10"=w612:bool)
    n391 = Not(x=w610) -> (.not. x?=w611:bool)
    n392 = And(x=w612, y=w611) -> (x .and. y?=w609:bool)
    n393 = Exclusive Or(1:w607, 2:w609) -> (0:w608:bool)
    n394 = case shown="False" w608 {
      tunnel: w616 -> [w619 w625]
      tunnel: w615 -> [w620 w624]
      frame False {
        n395 = call <vilib>:"WPI_MotorControlSetOutput.vi"("Output"=0.0, "MotorControlDevRef"=w619) -> ()  [unwired: 7 in, 3 out]
        n396 = call <vilib>:"WPI_MotorControlSetOutput.vi"("Output"=0.0, "MotorControlDevRef"=w620) -> ()  [unwired: 7 in, 3 out]
      }
      frame True {
        n397 = global read "Robot Global Data.vi" "Wingman Joystick"() -> (w623:T20)
        n398 = Unbundle By Name(w623) -> ("Button 4"=w622:bool)
        n399 = case shown="False" w622 {
          tunnel: w625 -> [w628 w630]
          tunnel: w624 -> [w629 w631]
          frame False {
            n400 = call <vilib>:"WPI_MotorControlSetOutput.vi"("Output"=1.0, "MotorControlDevRef"=w628) -> ()  [unwired: 7 in, 3 out]
            n401 = call <vilib>:"WPI_MotorControlSetOutput.vi"("Output"=-1.0, "MotorControlDevRef"=w629) -> ()  [unwired: 7 in, 3 out]
          }
          frame True {
            n402 = call <vilib>:"WPI_MotorControlSetOutput.vi"("Output"=1.0, "MotorControlDevRef"=w631) -> ()  [unwired: 7 in, 3 out]
            n403 = call <vilib>:"WPI_MotorControlSetOutput.vi"("Output"=-1.0, "MotorControlDevRef"=w630) -> ()  [unwired: 7 in, 3 out]
          }
        }
      }
    }
    n404 = Wait (ms)(milliseconds to wait=u32 20) -> ()  [unwired: 1 out]
  }
